vi "TDS_ConfigureTrigger.vi"(7 "instrument handle":refnum<k15>, 8 "error in":errorcluster, 11 "VI ServerCluster":T1) -> (0 "error out":errorcluster)   [LabVIEW 2020]
uses:
  LabVIEW 2020 Toolkits/VI Server Toolkit/VI Server_TypeDefs/VI Server_RefsCluster.ctl
  LabVIEW 2020 Toolkits/VI Server Toolkit/VI Server Libraries/VI Server_GetControl.llb/VI Server_STR_Get.vi
  LabVIEW 2020 Toolkits/VI Server Toolkit/VI Server Libraries/VI Server_GetControl.llb/VI Server_DBL_Get.vi
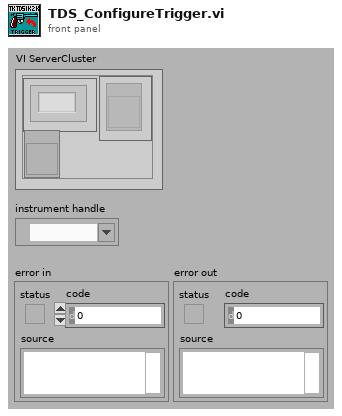
[diagram p1: front panel]
types:
  T1 = typedef "VI Server_RefsCluster.ctl" = cluster{"Labels":string[], "Refs":refnum<vi>[], "VI Ref":refnum<vi>}
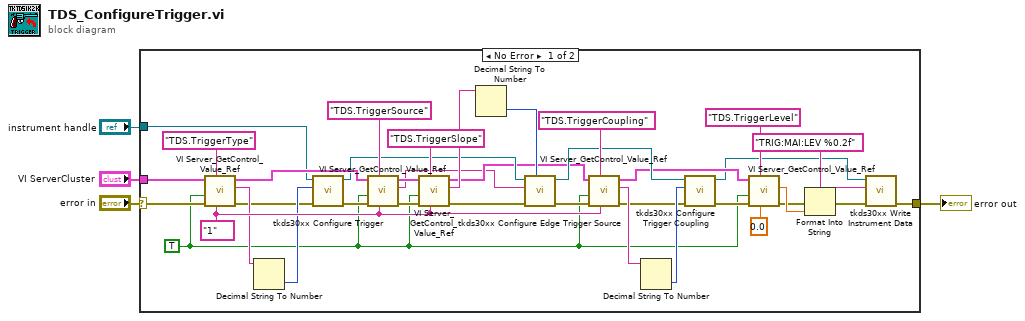
[diagram p0: block diagram]
diagram:
  n1 = case shown="No Error" "error in" {
    selector: "error in" -> [w20 w43]
    tunnel: [w8 w43] -> w4
    tunnel: "VI ServerCluster" -> [w21 _]
    tunnel: "instrument handle" -> [w22 _]
    frame No Error {
      w5 = TRUE ("SingleInstance")
      w42 = "1" ("Default Value")
      n2 = call-poly "VI Server_GetControl_Value_Ref.vi"("DataType"=w42, "Control.Label"="TDS.TriggerType" ("Label"), "error in"=w20, "SingleInstance"=w5, "VI Server.RefsCluster"=w21) -> ("error out"=w24:errorcluster, "Value"=w26:string, "VI Server.RefsCluster.DUP"=w29:T1)  [unwired: 3 in, 1 out]
      n3 = Decimal String To Number(string=w26) -> (number=w27:i32)  [unwired: 2 in, 1 out]
      n4 = call "tkds30xx Configure Trigger.vi"("error in (no error)"=w24, "Trigger Type (Edge)"=w27, "instrument handle"=w22) -> ("error out"=w28:errorcluster, "instrument handle out"=w23:refnum<k15>)  [unwired: 7 in]
      n5 = call-poly "VI Server_GetControl_Value_Ref.vi"("DataType"=w42, "Control.Label"="TDS.TriggerSource" ("Label"), "error in"=w28, "SingleInstance"=w5, "VI Server.RefsCluster"=w29) -> ("error out"=w31:errorcluster, "Value"=w17:string, "VI Server.RefsCluster.DUP"=w32:T1)  [unwired: 3 in, 1 out]
      n6 = call-poly "VI Server_GetControl_Value_Ref.vi"("DataType"=w42, "Control.Label"="TDS.TriggerSlope" ("Label"), "error in"=w31, "SingleInstance"=w5, "VI Server.RefsCluster"=w32) -> ("error out"=w18:errorcluster, "Value"=w34:string, "VI Server.RefsCluster.DUP"=w19:T1)  [unwired: 3 in, 1 out]
      n7 = Decimal String To Number(string=w34) -> (number=w35:i32)  [unwired: 2 in, 1 out]
      n8 = call "tkds30xx Configure Edge Trigger Source.vi"("Trigger Slope (Positive)"=w35, "error in (no error)"=w18, "Trigger Source (Channel 1)"=w17, "instrument handle"=w23) -> ("error out"=w37:errorcluster, "instrument handle out"=w36:refnum<k15>)  [unwired: 6 in]
      n9 = call-poly "VI Server_GetControl_Value_Ref.vi"("DataType"=w42, "Control.Label"="TDS.TriggerCoupling" ("Label"), "error in"=w37, "SingleInstance"=w5, "VI Server.RefsCluster"=w19) -> ("error out"=w38:errorcluster, "Value"=w40:string, "VI Server.RefsCluster.DUP"=w15:T1)  [unwired: 3 in, 1 out]
      n10 = Decimal String To Number(string=w40) -> (number=w41:i32)  [unwired: 2 in, 1 out]
      n11 = call "tkds30xx Configure Trigger Coupling.vi"("error in (no error)"=w38, "Trigger Coupling (Low Frequency Reject)"=w41, "instrument handle"=w36) -> ("error out"=w16:errorcluster, "instrument handle out"=w7:refnum<k15>)  [unwired: 7 in]
      n12 = call-poly "VI Server_GetControl_Value_Ref.vi"("DataType"=0.0, "Control.Label"="TDS.TriggerLevel" ("Label"), "error in"=w16, "SingleInstance"=w5, "VI Server.RefsCluster"=w15) -> ("error out"=w11:errorcluster, "Value"=w12:dbl)  [unwired: 3 in, 2 out]
      n13 = Format Into String(format string="TRIG:MAI:LEV %0.2f", error in=w11, w12) -> (resulting string=w6:string, error out=w9:errorcluster)  [unwired: 1 in]
      n14 = call "tkds30xx Write Instrument Data.vi"("error in (no error)"=w9, "Write Buffer"=w6, "instrument handle"=w7) -> ("error out"=w8:errorcluster)  [unwired: 7 in, 1 out]
    }
    frame Error {
    }
  }
  "error out" <- w4
